vi "Read String Comparator.vi"(8 "error in (no error)":errorcluster, 11 "String Assertion in":refnum<class "String Assertion.lvclass">) -> (0 "error out":errorcluster, 2 "String Comparator":T1, 3 "String Assertion out":refnum<class "String Assertion.lvclass">)   [LabVIEW 2020, in "MacroAssert.lvlib" / "String Assertion.lvclass"]
uses:
  String Assertion.lvclass
  String Comparator.ctl
  String Assertion.lvclass/String Assertion.ctl
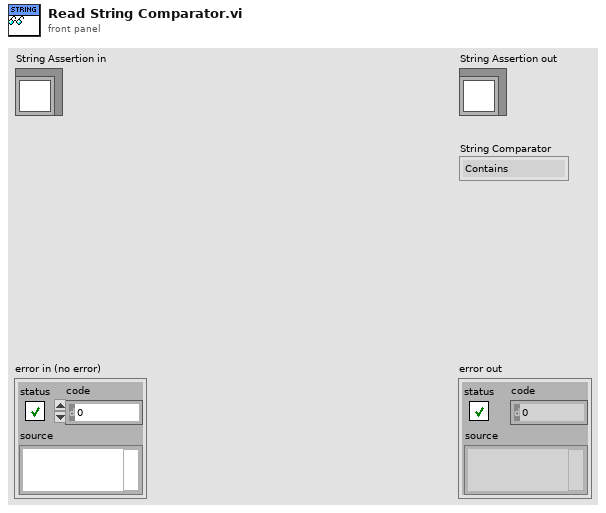
[diagram p1: front panel]
types:
  T1 = typedef "MacroAssert.lvlib/String Assertion.lvclass/String Comparator.ctl" = enum16{"Contains", "Equals", "Starts with", "Ends with", "Does not contain", "Does not equal"}
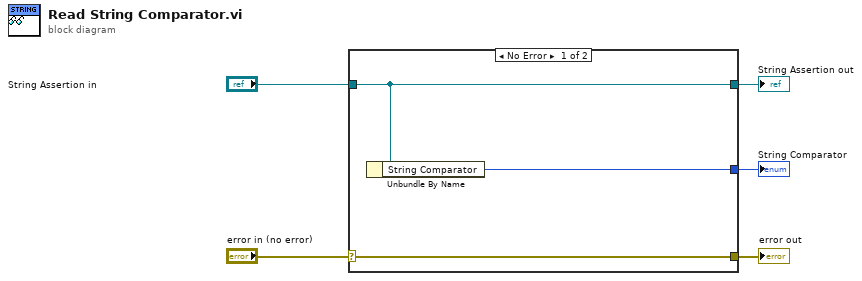
[diagram p0: block diagram]
diagram:
  n1 = case shown="No Error" "error in (no error)" {
    selector: "error in (no error)" -> [w8 w9]
    tunnel: [w8 w9] -> w4
    tunnel: [w7 w10] -> w2
    tunnel: "String Assertion in" -> [w7 w10]
    tunnel: [w6 _] -> w1
    frame No Error {
      n2 = Unbundle By Name(w7) -> ("String Comparator"=w6:T1)
    }
    frame Error {
    }
  }
  "error out" <- w4
  "String Assertion out" <- w2
  "String Comparator" <- w1
